vi "Destructor.vi"(8 "error in (no error)":errorcluster, 11 "Configuration in":refnum<class "Configuration.lvclass">) -> (0 "error out":errorcluster, 3 "Configuration out":refnum<class "Configuration.lvclass">)   [LabVIEW 2011, in "Configuration.lvclass"]
uses:
  Configuration.lvclass
  Configuration.lvclass/Configuration.ctl
  <vilib>/Utility/config.llb/Config Data RefNum.ctl
  <vilib>/Utility/config.llb/NI_LVConfig.lvlib
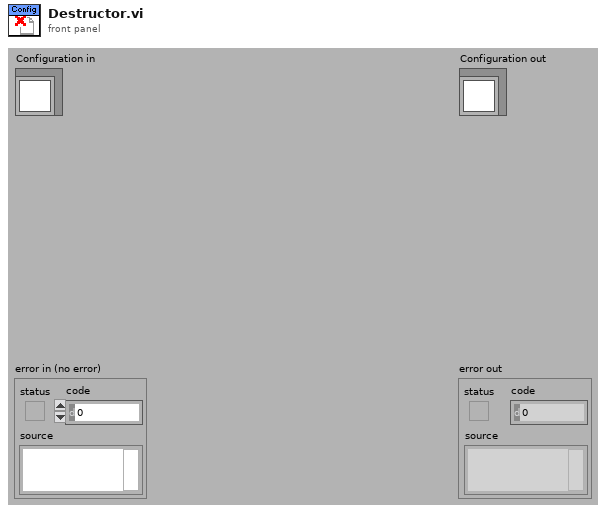
[diagram p1: front panel]
types:
  T1 = typedef "Configuration.lvclass/File Type.ctl" = enum16{"INI", "XML"}
  T2 = typedef "NI_LVConfig.lvlib/Config Data RefNum.ctl" = refnum<k1>
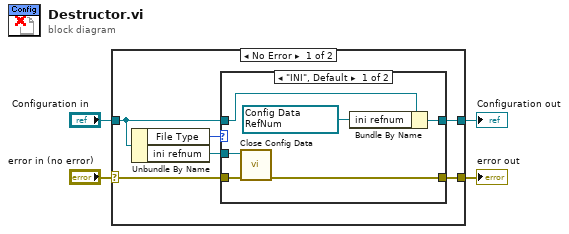
[diagram p0: block diagram]
diagram:
  n1 = case shown="No Error" "error in (no error)" {
    selector: "error in (no error)" -> [w8 w20]
    tunnel: [w7 w20] -> w3
    tunnel: [w9 w19] -> w1
    tunnel: "Configuration in" -> [w10 w19]
    frame No Error {
      n2 = Unbundle By Name(w10) -> ("File Type"=w6:T1, "ini refnum"=w5:T2)
      n3 = case shown="\"INI\", Default" w6 {
        tunnel: w10 -> [w16 w17]
        tunnel: [w14 w17] -> w9
        tunnel: w8 -> [w13 w18]
        tunnel: [w12 w18] -> w7
        tunnel: w5 -> [w11 _]
        frame "INI", Default {
          w15 = T2 refnum items=["config data"] ("refnum")
          n4 = call <vilib>:"Close Config Data.vi"("error in (no error)"=w13, "refnum"=w11) -> ("error out"=w12:errorcluster)  [unwired: 8 in, 1 out]
          n5 = Bundle By Name(cluster=w16, "ini refnum"=w15) -> (w14:refnum<class "Configuration.lvclass">)
        }
        frame "XML" {
        }
      }
    }
    frame Error {
    }
  }
  "error out" <- w3
  "Configuration out" <- w1
